vi "Create connection 2 (SubVI).vi"(2 "error in (no error)":errorcluster, 3 "host name":string, 4 "Connection in":refnum<class "Connection.lvclass">) -> (0 "error out":errorcluster, 1 "Connection out":refnum<class "Connection.lvclass">)   [LabVIEW 2016]
uses:
  <vilib>/Distrio/LabbitMQ/Connection/Connection.lvclass
  <vilib>/Distrio/LabbitMQ/Connection/connection_parameters_cluster.ctl
  global/AMQP_credentials.vi
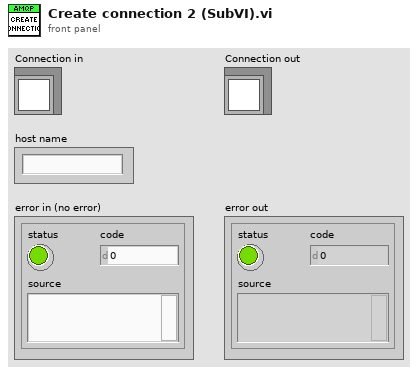
[diagram p1: front panel]
types:
  T1 = typedef "Connection.lvclass/connection_parameters_cluster.ctl" = cluster{"host name":string, "port":i32, "user name":string, "password":string, "virtual host":string}
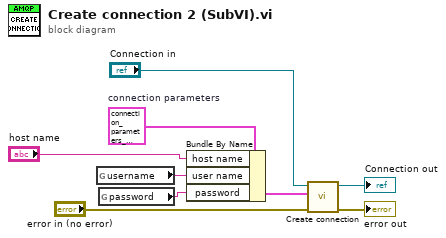
[diagram p0: block diagram]
diagram:
  w7 = T1 {"host name"="localhost", "port"=5672, "user name"="guest", "password"="guest", "virtual host"="/"}  # connection parameters
  n1 = global read "AMQP_credentials.vi" "username"() -> (w5:string)
  n2 = global read "AMQP_credentials.vi" "password"() -> (w4:string)
  n3 = Bundle By Name(cluster=w7, "host name"="host name", "user name"=w5, "password"=w4) -> (w6:T1)
  n4 = call <vilib>:"Create connection.vi"("error in (no error)"="error in (no error)", "connection parameters"=w6, "Connection in"="Connection in") -> ("error out"=→"error out":errorcluster, "Connection out"=→"Connection out":refnum<class "Connection.lvclass">)  [unwired: 7 in]
